vi "Get Properties.vi"(8 "error in (no error)":errorcluster, 11 "TDMS Log File Specification in":refnum<class "TDMS Log File Specification.lvclass">) -> (0 "error out":errorcluster, 2 "Properties":T1[](array[typedef]), 3 "TDMS Log File Specification out":refnum<class "TDMS Log File Specification.lvclass">)   [LabVIEW 2012, in "Waveform Data Logger Shared.lvlib" / "TDMS Log File Specification.lvclass"]
uses:
  TDMS Log File Specification.lvclass
  Property Specification.ctl
  TDMS Log File Specification.lvclass/TDMS Log File Specification.ctl
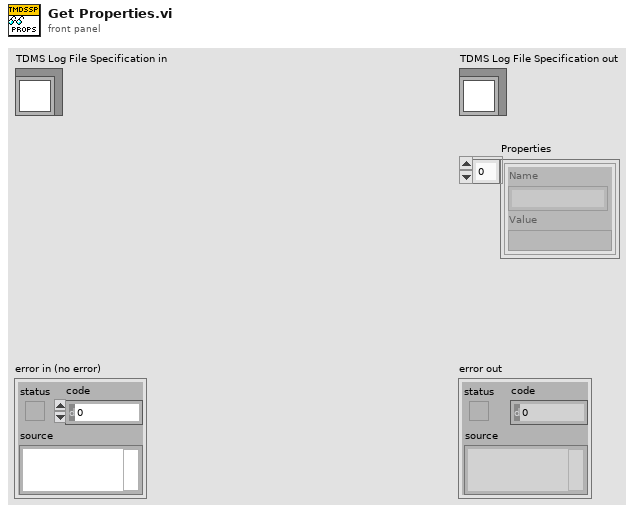
[diagram p1: front panel]
types:
  T1 = typedef "Waveform Data Logger Shared.lvlib/TDMS Log File Specification.lvclass/Property Specification.ctl" = cluster{"Name":string, "Value":variant}
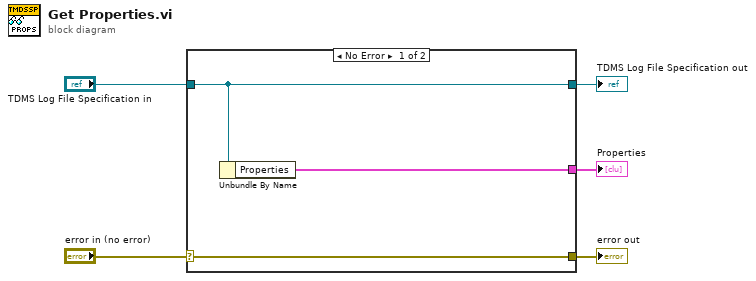
[diagram p0: block diagram]
diagram:
  n1 = case shown="No Error" "error in (no error)" {
    selector: "error in (no error)" -> [w8 w9]
    tunnel: [w8 w9] -> w4
    tunnel: [w7 w10] -> w2
    tunnel: "TDMS Log File Specification in" -> [w7 w10]
    tunnel: [w6 _] -> w1
    frame No Error {
      n2 = Unbundle By Name(w7) -> ("Properties"=w6:T1[])
    }
    frame Error {
    }
  }
  "error out" <- w4
  "TDMS Log File Specification out" <- w2
  "Properties" <- w1
